vi "DSF.Engine.Framework.Get Builder Manager.vi"(11 "Framework in":refnum<class "Framework.lvclass">) -> (2 "Builder Manager":refnum<class "DSF.Engine.BuilderManager.lvclass">, 3 "Framework out":refnum<class "Framework.lvclass">)   [LabVIEW 2017, in "DSF.Engine.lvlib" / "Framework.lvclass"]
uses:
  Framework.lvclass
  BuilderManager/DSF.Engine.BuilderManager.lvclass
  Framework.lvclass/Framework.ctl
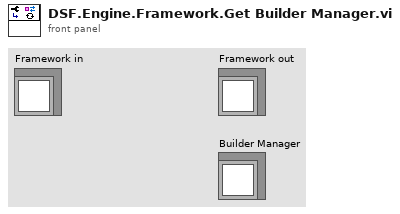
[diagram p1: front panel]
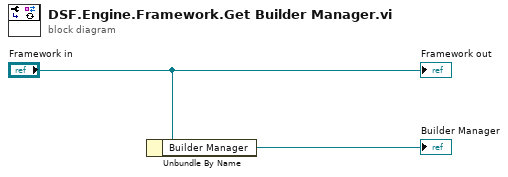
[diagram p0: block diagram]
diagram:
  n1 = Unbundle By Name("Framework in") -> ("Builder Manager"=→"Builder Manager":refnum<class "DSF.Engine.BuilderManager.lvclass">)
  "Framework out" <- "Framework in"
